vi "Is VI Server Required.vi"(8 "error in (no error)":errorcluster, 11 "Macro in":refnum<class "Macro.lvclass">) -> (0 "error out":errorcluster, 2 "VI Server Required?":bool, 3 "Macro out":refnum<class "Macro.lvclass">)   [LabVIEW 2020, in "MacroAssert.lvlib" / "Macro.lvclass"]
doc: "Outputs whether VI Server is required to perform the given macro."
uses:
  Macro.lvclass
  Step/Step.lvclass
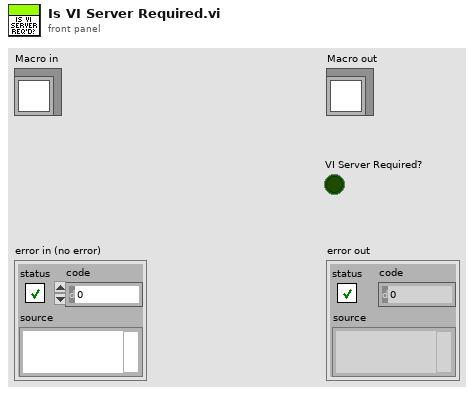
[diagram p1: front panel]
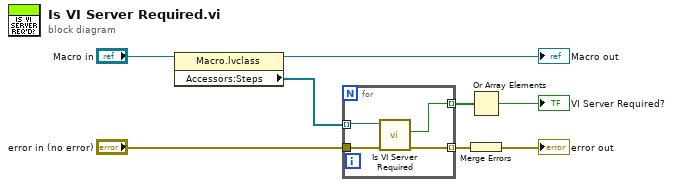
[diagram p0: block diagram]
diagram:
  n1 = property class="Macro.lvclass"(reference="Macro in") -> (reference out=→"Macro out":refnum<class "Macro.lvclass">, "Accessors:Steps"=w6:refnum<class "Step.lvclass">[])  [unwired: 1 in, 1 out]
  n2 = for {
    tunnel: w6 -> [w12] mode=indexing
    tunnel: "error in (no error)" -> [w11]
    tunnel: [w10] -> w4 mode=indexing
    tunnel: [w9] -> w2 mode=indexing
    n3 = call-dynamic "Is VI Server Required.vi"("error in (no error)"=w11, "Step in"=w12) -> ("error out"=w10:errorcluster, "VI Server Required?"=w9:bool)  [unwired: 7 in, 1 out]
  }
  n4 = Or Array Elements(Boolean array=w2) -> (logical OR=→"VI Server Required?":bool)
  n5 = Merge Errors(w4) -> (→"error out":errorcluster)
